vi "ConvertPotentiometerToDegrees.vi"(1 "Zero Position 1 [0,1]":dbl, 2 "Raw Potentiometer Value [0,1]":dbl) -> (0 "Orientation (deg) [-180, +180]":dbl)   [LabVIEW 2019]
doc: "Converts a potentiometer (or similar analog sensor) from a range of 0 to 1, to -180 degrees to +180 degrees. Supports a calibration value."
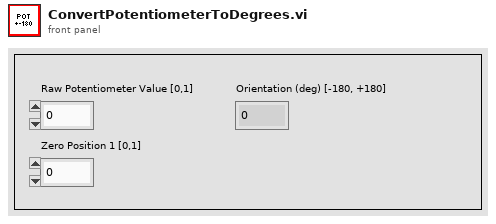
[diagram p1: front panel]
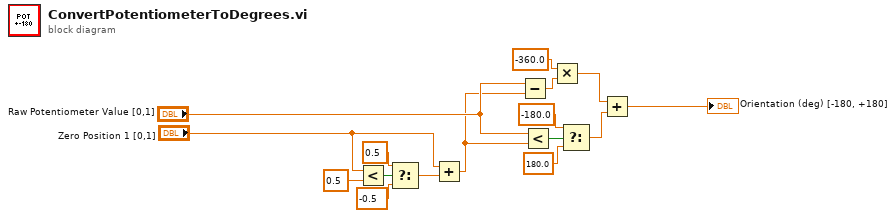
[diagram p0: block diagram]
diagram:
  n1 = Less?(x="Zero Position 1 [0,1]", y=0.5) -> (x < y?=w10:bool)
  n2 = Select(t=0.5 ("x"), s=w10, f=-0.5 ("x")) -> (s? t:f=w13:dbl)
  n3 = Add(x="Zero Position 1 [0,1]", y=w13) -> (x+y=w8:dbl)
  n4 = Subtract(x="Raw Potentiometer Value [0,1]", y=w8) -> (x-y=w2:dbl)
  n5 = Less?(x="Raw Potentiometer Value [0,1]", y=w8) -> (x < y?=w7:bool)
  n6 = Multiply(x=-360.0, y=w2) -> (x*y=w3:dbl)
  n7 = Select(t=-180.0, s=w7, f=180.0) -> (s? t:f=w4:dbl)
  n8 = Add(x=w3, y=w4) -> (x+y=→"Orientation (deg) [-180, +180]":dbl)
